vi "Both Mic Data seperately acquired_not changed.vi"() -> ()   [LabVIEW 2021]
panel:
  in  "rate":dbl=51200.0
  in  "number of samples":i32=10000
  out "Waveform Chart 2":dynamicdata(graph)
  out "Waveform Chart":dynamicdata(graph)
  in  "stop (F)":bool
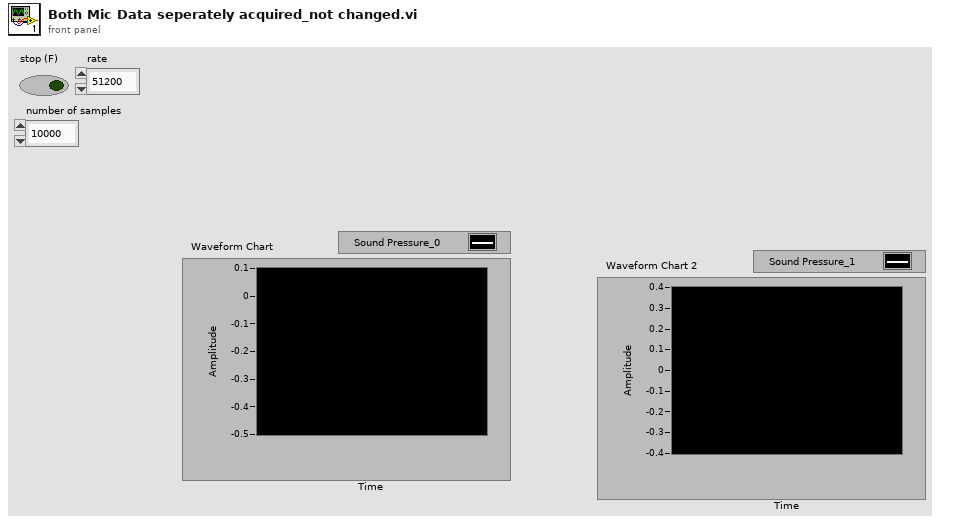
[diagram p1: front panel]
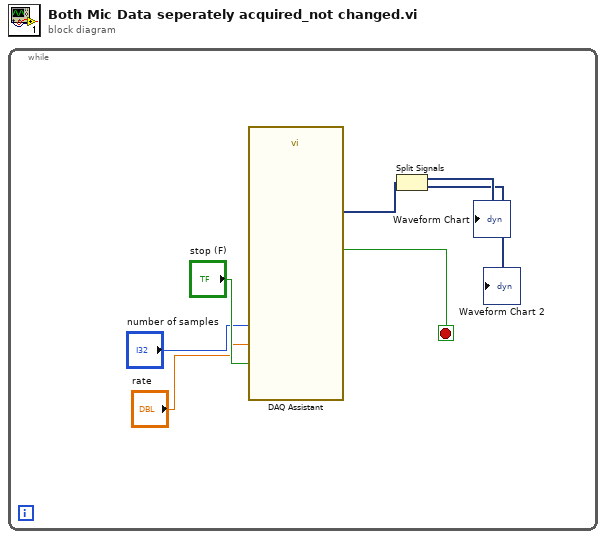
[diagram p0: block diagram]
diagram:
  n1 = while {
    stop <- w6 stop-if-true
    n2 = call "DAQ Assistant"("rate"="rate", "number of samples"="number of samples", "stop (F)"="stop (F)") -> ("data"=w3:dynamicdata, "stopped"=w6:bool)  [unwired: 13 in, 2 out]
    n3 = Split Signals(w3) -> (→"Waveform Chart":dynamicdata, →"Waveform Chart 2":dynamicdata)  [unwired: 2 in]
  }
